vi "test_Set FPGA Bitfile.vi"(8 "error in (no error)":errorcluster, 11 "TestCase in":refnum<class "FPGA Addon Scripting API Unit Tests.lvclass">) -> (0 "error out":errorcluster, 3 "TestCase out":refnum<class "FPGA Addon Scripting API Unit Tests.lvclass">)   [LabVIEW 2021, in "FPGA Addon Scripting API Unit Tests.lvclass"]
uses:
  FPGA Addon Scripting API Unit Tests.lvclass
  APIs/Scripting API/TypeDefs/Output Scalar Data.ctl
  Addon/Addon Shared/Types/FPGA Addon Data Type.ctl
  <vilib>/addons/_JKI Toolkits/VI Tester/TestCase.llb/TestCase.lvclass
  FPGA Addon Test Class/FPGA Addon Test Class.lvclass
  APIs/Scripting API/Scripting API.lvlib
  Addon/Addon Shared/FPGA Addon Shared.lvlib
  C:/Program Files/National Instruments/LabVIEW 2021/vi.lib/addons/_JKI Toolkits/VI Tester/TestCase.llb/TestCase.lvclass
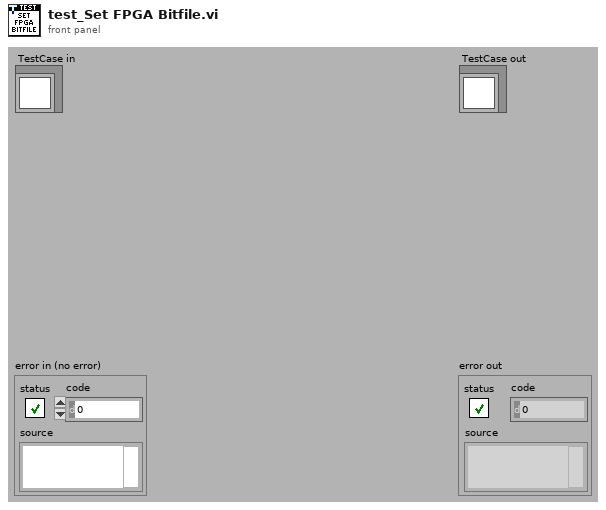
[diagram p1: front panel]
types:
  T1 = typedef "Scripting API.lvlib/Output Scalar Data.ctl" = cluster{"Bitfile Name":string, "SysDef Channel Name":string, "Imported":bool, "Data Type":T2}
  T2 = typedef "FPGA Addon Shared.lvlib/FPGA Addon Data Type.ctl" = enum8{"<Null>", "I8", "I16", "I32", "I64", "U8", "U16", "U32", "U64", "SGL", "Boolean", "Analog PWM In Settings", "Analog PWM In", "Digital PWM In Settings", "Digital PWM In", "Digital PWM Out", "Sine Out", "FXP", "FXP+/-24.5", "FXP+/-16.5", "FXP+/-32.8", "FXP+/-64.32", "FXP+/-16.7", "FXP+/-20.5", "FXP+/-27.5", "FXP+/-32.16", "FXP+16.3", "FXP+18.3", "Digital Static In", "Digital Static Out", "Digital Static In Settings", "Digital WSS Out", "Quad Encoder Settings", "Quad Encoder In", "Group"}
  T3 = typedef "Custom Device API.lvlib/Custom Device Item Ref.ctl" = u64
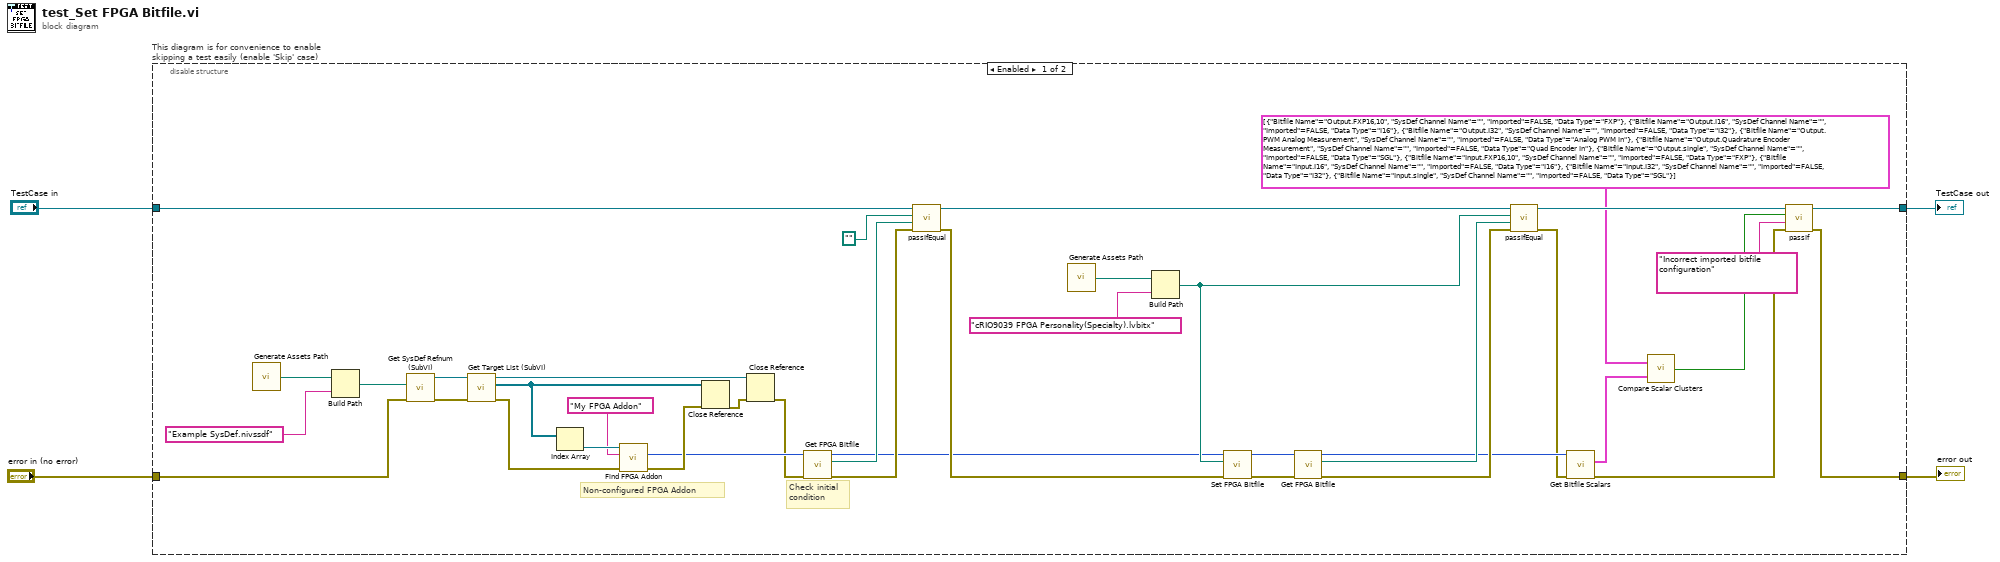
[diagram p0: block diagram]
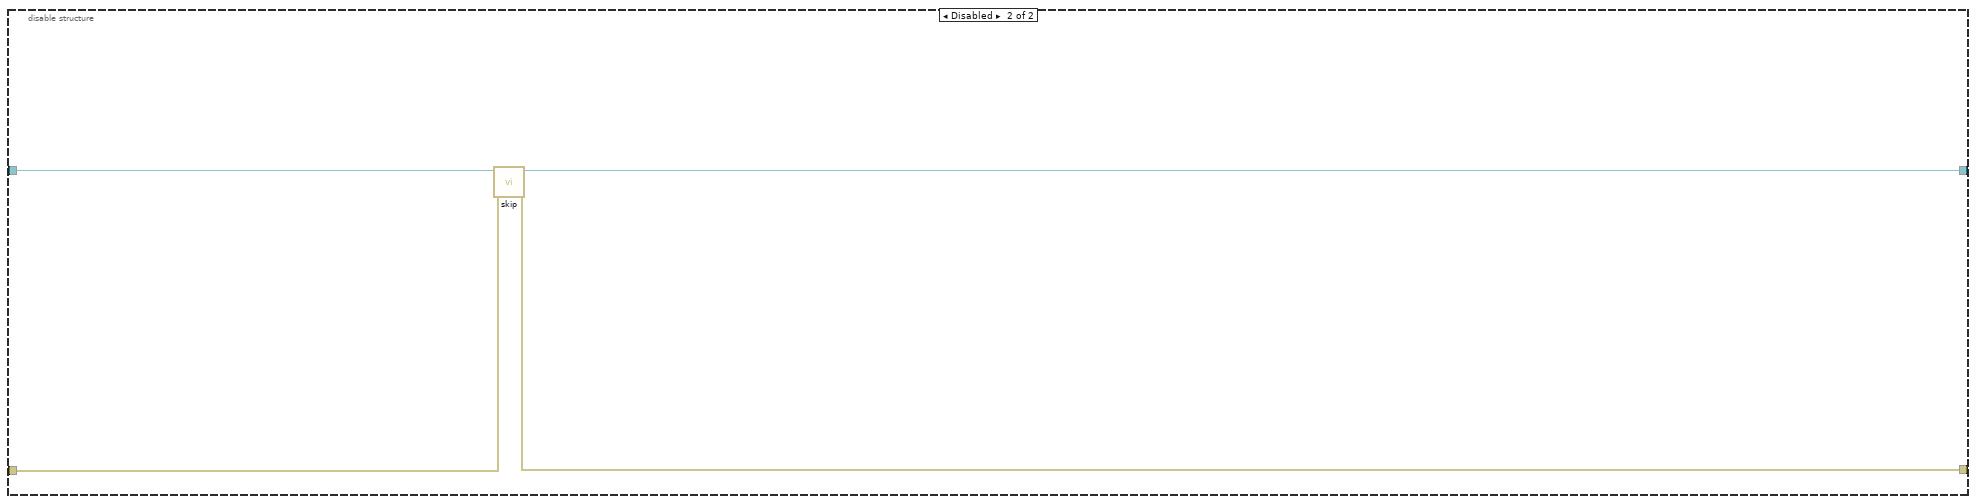
[diagram p2: hidden frame]
diagram:
  n1 = disable-structure "This diagram is for convenience to enable skipping a test easily (enable 'Skip' case)" shown="Enabled" {
    disable-tunnel: "TestCase in" -> [w21 w47]
    disable-tunnel: [w10 w45] -> w1
    disable-tunnel: [w7 w46] -> w3
    disable-tunnel: "error in (no error)" -> [w39 w44]
    frame Enabled {
      # "Check initial condition"
      # "Non-configured FPGA Addon"
      n2 = call "Generate Assets Path.vi"() -> ("Assets path"=w43:path)
      n3 = Build Path(base path=w43, name or relative path="Example SysDef.nivssdf") -> (appended path=w41:path)
      n4 = call "Get SysDef Refnum (SubVI).vi"("error in (no error)"=w39, "System Definition path"=w41) -> ("error out"=w38:errorcluster, "SysDef Refnum out"=w40:refnum<k24>)  [unwired: 8 in]
      n5 = call "Get Target List (SubVI).vi"("error in (no error)"=w38, "SysDef Refnum in"=w40) -> ("error out"=w33:errorcluster, "Target List Refnums"=w37:refnum<k24>[], "SysDef Refnum out"=w36:refnum<k24>)  [unwired: 7 in]
      n6 = Index Array(array=w37) -> (element=w34:refnum<k24>)  [unwired: 1 in]
      n7 = call "Find FPGA Addon.vi"("error in"=w33, "FPGA addon name"="My FPGA Addon", "target in"=w34) -> ("error out"=w31:errorcluster, "FPGA addon refnum out"=w23:T3)  [unwired: 5 in, 2 out]
      n8 = Close Reference(reference=w37, error in (no error)=w31) -> (error out=w35:errorcluster)
      n9 = Close Reference(reference=w36, error in (no error)=w35) -> (error out=w22:errorcluster)
      n10 = call "Get FPGA Bitfile.vi"("error in"=w22, "FPGA addon refnum in"=w23) -> ("error out"=w18:errorcluster, "FPGA bitfile path"=w19:path, "FPGA addon refnum out"=w15:T3)  [unwired: 7 in]
      n11 = call-dynamic "passIfEqual.vi"("error in (no error)"=w18, "y"=w19, "x"=path "", "TestCase in"=w21) -> ("error out"=w17:errorcluster, "TestCase out"=w20:refnum<class "FPGA Addon Scripting API Unit Tests.lvclass">)  [unwired: 6 in]
      n12 = call "Generate Assets Path.vi"() -> ("Assets path"=w30:path)
      n13 = Build Path(base path=w30, name or relative path="cRIO9039 FPGA Personality(Specialty).lvbitx") -> (appended path=w24:path)
      n14 = call "Set FPGA Bitfile.vi"("error in"=w17, "FPGA bitfile path"=w24, "FPGA addon refnum in"=w15) -> ("error out"=w26:errorcluster, "FPGA addon refnum out"=w25:T3)  [unwired: 7 in]
      n15 = call "Get FPGA Bitfile.vi"("error in"=w26, "FPGA addon refnum in"=w25) -> ("error out"=w27:errorcluster, "FPGA bitfile path"=w28:path, "FPGA addon refnum out"=w14:T3)  [unwired: 7 in]
      n16 = call-dynamic "passIfEqual.vi"("error in (no error)"=w27, "y"=w28, "x"=w24, "TestCase in"=w20) -> ("error out"=w13:errorcluster, "TestCase out"=w11:refnum<class "FPGA Addon Scripting API Unit Tests.lvclass">)  [unwired: 6 in]
      n17 = call "Get Bitfile Scalars.vi"("error in"=w13, "FPGA addon refnum in"=w14) -> ("error out"=w8:errorcluster, "bitfile scalars out"=w12:T1[])  [unwired: 7 in, 1 out]
      n18 = call "Compare Scalar Clusters.vi"("Target bitfile scalars in"=w12, "Reference bitfile scalars in"=T1[] [{"Bitfile Name"="Output.FXP16,10", "SysDef Channel Name"="", "Imported"=FALSE, "Data Type"=enum."FXP"}, {"Bitfile Name"="Output.I16", "SysDef Channel Name"="", "Imported"=FALSE, "Data Type"=enum."I16"}, {"Bitfile Name"="Output.I32", "SysDef Channel Name"="", "Imported"=FALSE, "Data Type"=enum."I32"}, {"Bitfile Name"="Output.PWM Analog Measurement", "SysDef Channel Name"="", "Imported"=FALSE, "Data Type"=enum."Analog PWM In"}, {"Bitfile Name"="Output.Quadrature Encoder Measurement", "SysDef Channel Name"="", "Imported"=FALSE, "Data Type"=enum."Quad Encoder In"}, {"Bitfile Name"="Output.single", "SysDef Channel Name"="", "Imported"=FALSE, "Data Type"=enum."SGL"}, {"Bitfile Name"="Input.FXP16,10", "SysDef Channel Name"="", "Imported"=FALSE, "Data Type"=enum."FXP"}, {"Bitfile Name"="Input.I16", "SysDef Channel Name"="", "Imported"=FALSE, "Data Type"=enum."I16"}, {"Bitfile Name"="Input.I32", "SysDef Channel Name"="", "Imported"=FALSE, "Data Type"=enum."I32"}, {"Bitfile Name"="Input.single", "SysDef Channel Name"="", "Imported"=FALSE, "Data Type"=enum."SGL"}] ("bitfile scalars out")) -> ("Equal ?"=w9:bool)
      n19 = call-dynamic "passIf.vi"("error in (no error)"=w8, "message (\"\")"="Incorrect imported bitfile configuration" ("message (\"\")"), "pass"=w9, "TestCase in"=w11) -> ("error out"=w7:errorcluster, "TestCase out"=w10:refnum<class "FPGA Addon Scripting API Unit Tests.lvclass">)  [unwired: 6 in]
    }
    frame Disabled {
      # "skip test result while test is under development"
      n20 = call <vilib>:"skip.vi"("error in (no error)"=w44, "TestCase in"=w47) -> ("error out"=w46:errorcluster, "TestCase out"=w45:refnum<class "FPGA Addon Scripting API Unit Tests.lvclass">)  [unwired: 8 in]
    }
  }
  "error out" <- w3
  "TestCase out" <- w1
